vi "Untitled 2 (SubVI).vi"(11 "swerve modules":T4[](array[typedef])=[{"descr"="FR", "V"=0.0, "angle"=0.0, "POS target"=0.0, "POS last"=0.0, "POS delta"=0.0, "turn CW"=FALSE, "-R?"=FALSE, "from pivot to module"={"Rcg"=0.0, "theta cg (deg)"=0.0}, "wrt geom CTR"={"delX"=0, "delY"=0}, "coord wrt geom CTR"={"geomX"=0.0, "geomY"=0.0}, "corner wt (lbm)"=0.0}, {"descr"="FL", "V"=0.0, "angle"=0.0, "POS target"=0.0, "POS last"=0.0, "POS delta"=0.0, "turn CW"=FALSE, "-R?"=FALSE, "from pivot to module"={"Rcg"=0.0, "theta cg (deg)"=0.0}, "wrt geom CTR"={"delX"=0, "delY"=0}, "coord wrt geom CTR"={"geomX"=0.0, "geomY"=0.0}, "corner wt (lbm)"=0.0}, {"descr"="RL", "V"=0.0, "angle"=0.0, "POS target"=0.0, "POS last"=0.0, "POS delta"=0.0, "turn CW"=FALSE, "-R?"=FALSE, "from pivot to module"={"Rcg"=0.0, "theta cg (deg)"=0.0}, "wrt geom CTR"={"delX"=0, "delY"=0}, "coord wrt geom CTR"={"geomX"=0.0, "geomY"=0.0}, "corner wt (lbm)"=0.0}, {"descr"="RR", "V"=0.0, "angle"=0.0, "POS target"=0.0, "POS last"=0.0, "POS delta"=0.0, "turn CW"=FALSE, "-R?"=FALSE, "from pivot to module"={"Rcg"=0.0, "theta cg (deg)"=0.0}, "wrt geom CTR"={"delX"=0, "delY"=0}, "coord wrt geom CTR"={"geomX"=0.0, "geomY"=0.0}, "corner wt (lbm)"=0.0}] {"corner wt (lbm)" format="%.4g"; "angle" format="%.3g"; "coord wrt geom CTR"."geomY" format="%.4g"; "coord wrt geom CTR"."geomX" format="%.4g"; "from pivot to module"."theta cg (deg)" format="%.4g"; "from pivot to module"."Rcg" format="%.4g"; "POS delta" format="%.3g"; "POS last" format="%.3g"; "POS target" format="%.3g"; "V" format="%.3g"}) -> ()   [LabVIEW 2023]
uses:
  ctrl defs/ctrl swerve module.ctl
  ctrl defs/ctrl robot swerve dims.ctl
  ctrl defs/ctrl robot CG.ctl
  <vilib>/Analysis/coordinate.llb/Angle Units.ctl
  <vilib>/Analysis/coordinate.llb/Angle Range (Degree).ctl
  <vilib>/Analysis/coordinate.llb/Wrap Angle (scalar).vi
  <vilib>/Analysis/coordinate.llb/2D Cartesian Coordinate Shift (Scalar).vi
  Global INIT.vi
  <vilib>/Analysis/NI_AALPro.lvlib
  <vilib>/Analysis/NI_AAL_Angle.lvlib
  ctrl defs/ctrl XY coord.ctl
panel:
  out "CCW rotation angle":dbl[](array[numeric])
  out "angle from +X at CG ctr to wheel module":dbl[](array[numeric])
  out "angle from +X at geom ctr to wheel module":dbl[](array[numeric])
  out "ROBOT CG":T1={"mass (lbm)"=150.0, "CG"={"X"=24.0, "Y"=0.0}, "Zcg"=24.0} {"CG"."Y" format="%.4g"; "CG"."X" format="%.4g"}
  out "geom Y":dbl[](array[numeric])
  out "geom X":dbl[](array[numeric])
  out "ROBOT swerve dims":T3={"drive track"=24.428, "drive base"=24.428, "wheel  (in)"=4.0, "steer ratio"=21.42857, "drive ratio"=6.75, "enc ratio"=1.0}
  out "X Out":dbl[](array[numeric])
  out "Y Out":dbl[](array[numeric])
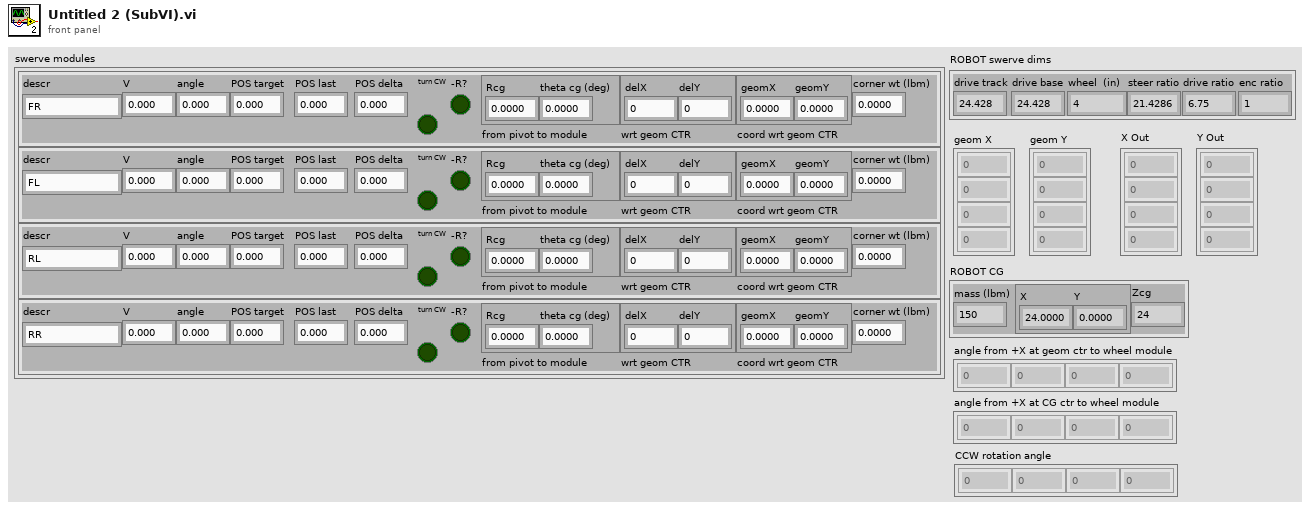
[diagram p1: front panel]
types:
  T1 = typedef "ctrl robot CG.ctl" = cluster{"mass (lbm)":dbl, "CG":T2, "Zcg":dbl}
  T2 = typedef "ctrl XY coord.ctl" = cluster{"X":dbl, "Y":dbl}
  T3 = typedef "ctrl robot swerve dims.ctl" = cluster{"drive track":dbl, "drive base":dbl, "wheel  (in)":dbl, "steer ratio":dbl, "drive ratio":dbl, "enc ratio":dbl}
  T4 = typedef "ctrl swerve module.ctl" = cluster{"descr":string, "V":dbl, "angle":dbl, "POS target":dbl, "POS last":dbl, "POS delta":dbl, "turn CW":bool, "-R?":bool, "from pivot to module":cluster{"Rcg":dbl, "theta cg (deg)":dbl}, "wrt geom CTR":cluster{"delX":i8, "delY":i8}, "coord wrt geom CTR":cluster{"geomX":dbl, "geomY":dbl}, "corner wt (lbm)":dbl}
  T5 = typedef "NI_AAL_Angle.lvlib/Angle Range (Degree).ctl" = u16
  T6 = typedef "NI_AAL_Angle.lvlib/Angle Units.ctl" = i32
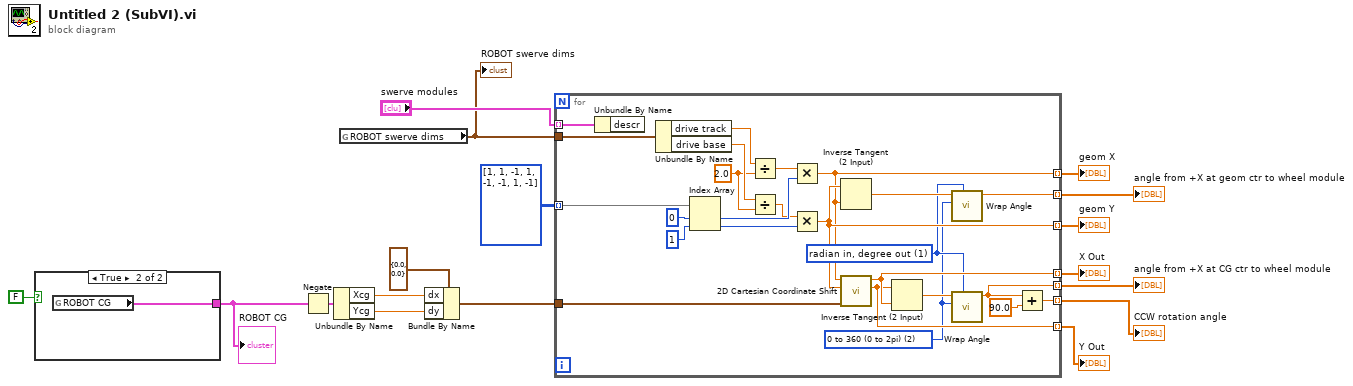
[diagram p0: block diagram]
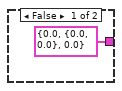
[diagram p2: hidden frame]
diagram:
  n1 = case shown="True" FALSE {
    tunnel: [T1 {"mass (lbm)"=0.0, "CG"={"X"=0.0, "Y"=0.0}, "Zcg"=0.0} ("ROBOT CG") w19] -> w10
    frame False {
    }
    frame True {
      n2 = global read "Global INIT.vi" "ROBOT CG"() -> (w19:T1)
    }
  }
  "ROBOT CG" <- w10
  n3 = Negate(x=w10) -> (-x=w9:T1)
  n4 = Unbundle By Name(w9) -> ("Xcg"=w8:dbl, "Ycg"=w7:dbl)
  n5 = global read "Global INIT.vi" "ROBOT swerve dims"() -> (w16:T3)
  "ROBOT swerve dims" <- w16
  n6 = Bundle By Name(cluster=cluster{"dx":dbl, "dy":dbl} {"dx"=0.0, "dy"=0.0} ("shift"), "dx"=w8, "dy"=w7) -> (w13:cluster{"dx":dbl, "dy":dbl})
  n7 = for {
    tunnel: "swerve modules" -> [w44] mode=indexing
    tunnel: w16 -> [w43]
    tunnel: i8[][] [[1, 1], [-1, 1], [-1, -1], [1, -1]] -> [w42] mode=indexing
    tunnel: w13 -> [w41]
    tunnel: [w30] -> w12 mode=indexing
    tunnel: [w31] -> w11 mode=indexing
    tunnel: [w25] -> w6 mode=indexing
    tunnel: [w26] -> w5 mode=indexing
    tunnel: [w28] -> w3 mode=indexing
    tunnel: [w24] -> w2 mode=indexing
    tunnel: [w22] -> w1 mode=indexing
    w20 = T5 2 items=["none", "-180 to 180 (-pi to pi)", "0 to 360 (0 to 2pi)"] ("angle range")
    w21 = T6 1 items=["radian in, radian out", "radian in, degree out", "degree in, degree out", "degree in, radian out"] ("angle units")
    w38 = 2.0 ("y")
    n8 = Unbundle By Name(w44) -> ()  [unwired: 1 out]
    n9 = Unbundle By Name(w43) -> ("drive track"=w40:dbl, "drive base"=w39:dbl)
    n10 = Index Array(array=w42, index #1=0 ("index"), index #2=1 ("index")) -> (element #1=w34:i8, element #2=w32:i8)
    n11 = Divide(x=w40, y=w38) -> (x/y=w35:dbl)
    n12 = Divide(x=w39, y=w38) -> (x/y=w33:dbl)
    n13 = Multiply(x=w35, y=w34) -> (x*y=w30:dbl)
    n14 = Multiply(x=w33, y=w32) -> (x*y=w31:dbl)
    n15 = Inverse Tangent (2 Input)(1:w30, 2:w31) -> (0:w29:dbl)
    n16 = call-poly <vilib>:"2D Cartesian Coordinate Shift.vi"("shift"=w41, "y"=w31, "x"=w30) -> ("y out"=w25:dbl, "x out"=w26:dbl)  [unwired: 6 in, 1 out]
    n17 = Inverse Tangent (2 Input)(1:w26, 2:w25) -> (0:w27:dbl)
    n18 = call-poly <vilib>:"Wrap Angle.vi"("angle units"=w21, "angle range"=w20, "angle in"=w29) -> ("angle out"=w28:dbl)  [unwired: 7 in, 1 out]
    n19 = call-poly <vilib>:"Wrap Angle.vi"("angle units"=w21, "angle range"=w20, "angle in"=w27) -> ("angle out"=w24:dbl)  [unwired: 7 in, 1 out]
    n20 = Add(x=w24, y=90.0) -> (x+y=w22:dbl)
  }
  "Y Out" <- w6
  "X Out" <- w5
  "geom X" <- w12
  "geom Y" <- w11
  "angle from +X at geom ctr to wheel module" <- w3
  "angle from +X at CG ctr to wheel module" <- w2
  "CCW rotation angle" <- w1
